vi "Create.vi"(9 "Alias":string, 10 "Actor":refnum<class "Actor.lvclass">, 11 "Base Actor in":refnum<class "Base Actor.lvclass">) -> (3 "Base Actor out":refnum<class "Base Actor.lvclass">)   [LabVIEW 2020, in "jettl.lvlib" / "Actor.lvlib" / "Base Actor.lvclass"]
uses:
  Base Actor.lvclass
  Actor/Actor.lvclass
  Attributes/Attributes/Attributes.lvclass
  Base Actor.lvclass/Base Actor.ctl
  Actor.lvlib
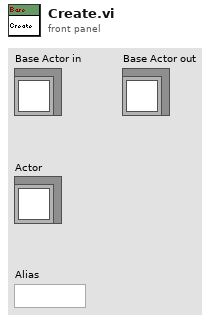
[diagram p1: front panel]
types:
  T1 = typedef "jettl.lvlib/Actor.lvlib/Created Aliases.ctl" = set{string}
  T2 = typedef "jettl.lvlib/Actor.lvlib/Created Attributes Map.ctl" = map{string, refnum<class "Attributes.lvclass">}
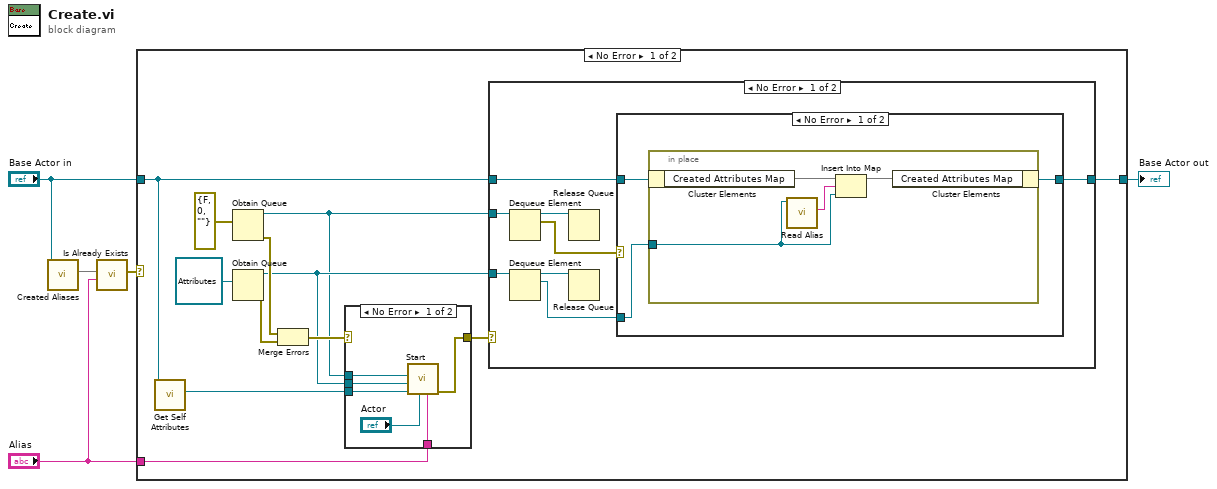
[diagram p0: block diagram]
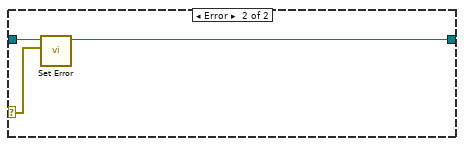
[diagram p2: hidden frame]
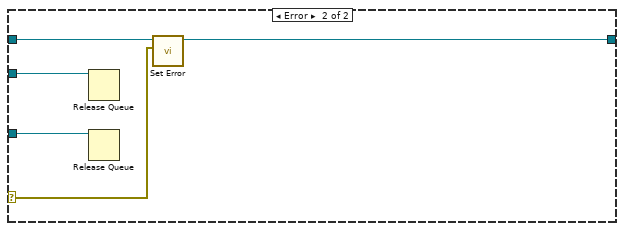
[diagram p3: hidden frame]
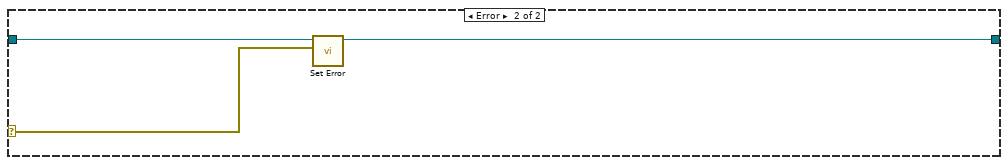
[diagram p5: hidden frame]
diagram:
  n1 = call-dynamic "Created Aliases.vi"("Base Actor in"="Base Actor in") -> ("Created Aliases"=w1:T1)  [unwired: 10 in]
  n2 = call "Is Already Exists.vi"("Alias"="Alias", "Created Aliases"=w1) -> ("Error"=w4:errorcluster)  [unwired: 9 in]
  n3 = case shown="No Error" w4 {
    selector: w4 -> [_ w48]
    tunnel: "Base Actor in" -> [w13 w50]
    tunnel: "Alias" -> [w16 _]
    tunnel: [w17 w49] -> w5
    frame No Error {
      n4 = call-dynamic "Get Self Attributes.vi"("Base Actor in"=w13) -> ("Self Attributes"=w12:refnum<class "Attributes.lvclass">)  [unwired: 10 in]
      n5 = Obtain Queue(element data type=errorcluster {"status"=FALSE, "code"=0, "source"=""} ("Error")) -> (queue out=w6:refnum<queue>, error out=w8:errorcluster)  [unwired: 4 in, 1 out]
      n6 = Obtain Queue(element data type=refnum<class "Attributes.lvclass"> refnum ("jettl.lvlib:Attributes.lvlib:Attributes.lvclass")) -> (queue out=w7:refnum<queue>, error out=w15:errorcluster)  [unwired: 4 in, 1 out]
      n7 = Merge Errors(w8, w15) -> (w9:errorcluster)
      n8 = case shown="No Error" w9 {
        selector: w9 -> [_ w47]
        tunnel: w16 -> [w45 _]
        tunnel: w12 -> [w43 _]
        tunnel: w7 -> [w42 _]
        tunnel: [w46 w47] -> w14
        tunnel: w6 -> [w41 _]
        frame No Error {
          n9 = call "Start.vi"("Alias"=w45, "Actor"="Actor", "Creator Attributes"=w43, "Queue of Self Attributes"=w42, "Queue of Error"=w41) -> ("Error"=w46:errorcluster)  [unwired: 6 in]
        }
        frame Error {
        }
      }
      n10 = case shown="No Error" w14 {
        selector: w14 -> [_ w37]
        tunnel: w13 -> [w25 w39]
        tunnel: [w24 w38] -> w17
        tunnel: w7 -> [w23 w40]
        tunnel: w6 -> [w21 w36]
        frame No Error {
          n11 = Dequeue Element(queue=w21) -> (queue out=w20:refnum<queue>, element=w18:errorcluster)  [unwired: 2 in, 2 out]
          n12 = Dequeue Element(queue=w23) -> (queue out=w22:refnum<queue>, element=w19:refnum<class "Attributes.lvclass">)  [unwired: 2 in, 2 out]
          n13 = Release Queue(queue=w20) -> ()  [unwired: 2 in, 3 out]
          n14 = Release Queue(queue=w22) -> ()  [unwired: 2 in, 3 out]
          n15 = case shown="No Error" w18 {
            selector: w18 -> [_ w33]
            tunnel: w25 -> [w27 w35]
            tunnel: [w26 w34] -> w24
            tunnel: w19 -> [w28 _]
            frame No Error {
              n16 = in-place {
                in-place-border: w28 -> [w29]
                n17 = in-place-cluster #1(w27) -> ("Created Attributes Map"=w32:T2)
                n18 = call-dynamic "Read Alias.vi"("Attributes in"=w29) -> ("Alias"=w30:string)  [unwired: 10 in]
                n19 = Insert Into Map(map in=w32, key=w30, value=w29) -> (map out=w31:T2)  [unwired: 2 out]
                n20 = in-place-cluster #1("Created Attributes Map"=w31) -> (w26:refnum<class "Base Actor.lvclass">)
              }
            }
            frame Error {
              n21 = call-dynamic "Set Error.vi"("Error"=w33, "Base Actor in"=w35) -> ("Base Actor out"=w34:refnum<class "Base Actor.lvclass">)  [unwired: 9 in]
            }
          }
        }
        frame Error {
          n22 = Release Queue(queue=w36) -> ()  [unwired: 2 in, 3 out]
          n23 = Release Queue(queue=w40) -> ()  [unwired: 2 in, 3 out]
          n24 = call-dynamic "Set Error.vi"("Error"=w37, "Base Actor in"=w39) -> ("Base Actor out"=w38:refnum<class "Base Actor.lvclass">)  [unwired: 9 in]
        }
      }
    }
    frame Error {
      n25 = call-dynamic "Set Error.vi"("Error"=w48, "Base Actor in"=w50) -> ("Base Actor out"=w49:refnum<class "Base Actor.lvclass">)  [unwired: 9 in]
    }
  }
  "Base Actor out" <- w5
